vi "EOL CAN_Clear_DTC's.vi"(11 "CAN Network ObjHandle":T1) -> (2 "TxRx Data":string[][](array[string]), 3 "Response Good?":bool)   [LabVIEW 2014]
uses:
  <vilib>/nican/nican.llb/xobjhandle.ctl
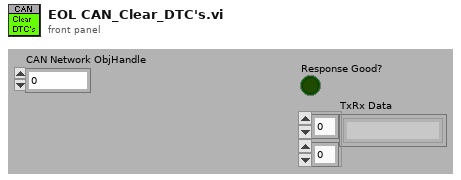
[diagram p1: front panel]
types:
  T1 = typedef "xobjhandle.ctl" = u32
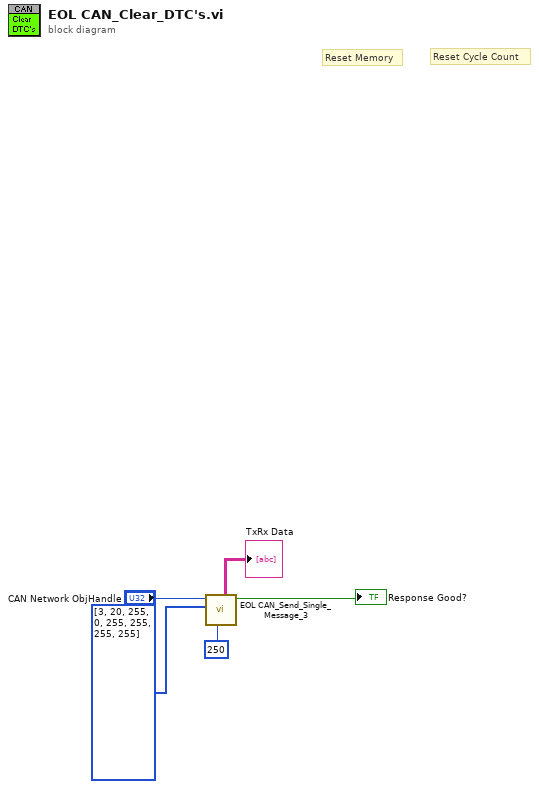
[diagram p0: block diagram]
diagram:
  # "Reset Memory"
  # "Reset Cycle Count"
  n1 = call <userlib>:"EOL CAN_Send_Single_Message_3.vi"("Msg Wait Time"=u32 250, "Tx Msg"=u8[] [3, 20, 255, 0, 255, 255, 255, 255] ("Transmit Data 2"), "NetworkObjHandle"="CAN Network ObjHandle") -> ("Response Good?"=→"Response Good?":bool, "TxRx Data"=→"TxRx Data":string[][])  [unwired: 5 in, 2 out]
